vi "Enqueue Message with Data.vi"(8 "error in (no error)":errorcluster, 9 "extra data":string, 10 "message ID":string, 11 "queue in":refnum<queue>) -> (0 "error out":errorcluster, 3 "queue out":refnum<queue>)   [LabVIEW 2020]
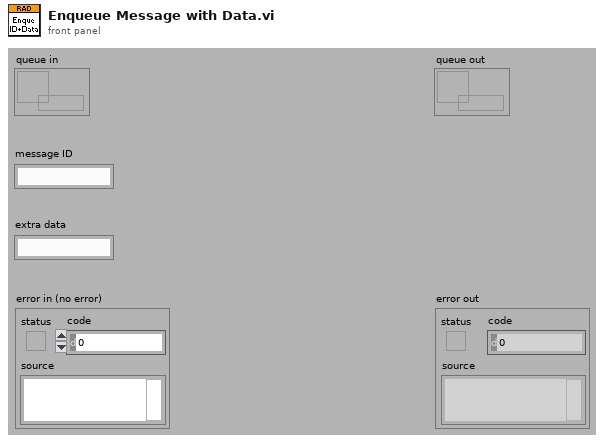
[diagram p1: front panel]
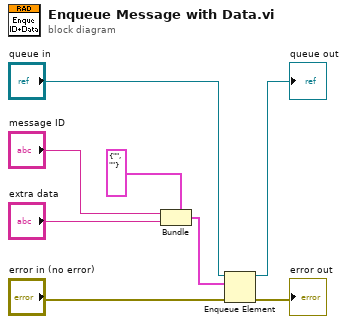
[diagram p0: block diagram]
diagram:
  n1 = Bundle(cluster=cluster{string, string} {"", ""}, "message ID", "extra data") -> (w1:cluster{string, string})
  n2 = Enqueue Element(queue="queue in", element=w1, error in (no error)="error in (no error)") -> (queue out=→"queue out":refnum<queue>, error out=→"error out":errorcluster)  [unwired: 1 in, 1 out]
